vi "SR830Monitor-new2.vi"() -> ()   [LabVIEW 2016]
doc: "This VI is an example of storing and recovering data from the SR830 data buffers .\nDATA STORAGE RATE specifes the rate at which data is added to the data buffers .\nSCAN LENGTH specifies the approximate length of the data acquisition scan is seconds .\nPLOT GRAPH, PLOT CH 1 DATA and PLOT CH 2 DATA specify if the respective graphs will be displayed .\nAfter data storage is completed , the channel 1 and channel 2 points are downloaded from the instrument to the CH 1 POINTS and CH 2 POINTS arrays respectively . \nSince data recovered (using the SR830 receive message.vi) is in the string format , this VI requires a considerable amount of time to format the data into an array of floating point numbers . A quicker way would be to store the string in a file and use a CIN to speed up the process ."
uses:
  Global/Global Variables/Data_Display_global.vi
  Instrument_Setup.vi
  Utility/Monitor Communication/sub-vis/SR830_Open_Queue.vi
  Utility/Monitor Communication/sub-vis/SR830_Check_Queue.vi
  Utility/Monitor Communication/SR830/SR830-Cluster.ctl
panel:
  out "SR830":T1={"Lockin 1"=[], "X1"=0.0, "Y1"=0.0, "X1 Percent"=0.0, "X1 Overload"=FALSE, "Y1 Overload"=FALSE, "Unit X1"="nV", "Unit X2"="nV", "Unit X2a"="nV", "Unit X1a"="nV", "Sensitivity Setpoint"=26, "X1 Percent 2"=0.0} {"X1 Percent 2" scale=0.0..1.0; "Sensitivity Setpoint" items=["2 nV", "5 nV", "10 nV", "20 nV", "50 nV", "100 nV", "200 nV", "500 nV", "1 µV", "2 µV", "5 µV", "10 µV", "20 µV", "50 µV", "100 µV", "200 µV", "500 µV", "1 mV", "2 mV", "5 mV", "10 mV", "20 mV", "50 mV", "100 mV", "200 mV", "500 mV", "1 V", ""]; "X1 Percent" scale=0.0..1.0; "X1" format="%#4_5f"}
  in  "Stopp":bool
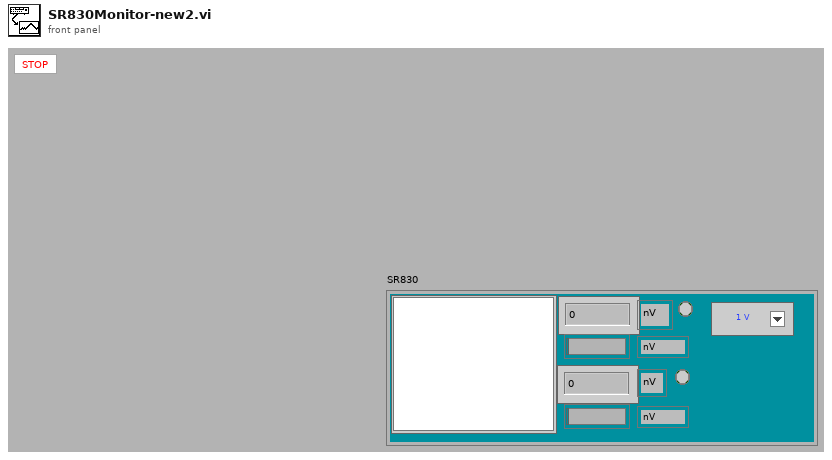
[diagram p1: front panel]
types:
  T1 = typedef "SR830-Cluster.ctl" = cluster{"Lockin 1":dbl[][], "X1":dbl, "Y1":dbl, "X1 Percent":dbl, "X1 Overload":bool, "Y1 Overload":bool, "Unit X1":string, "Unit X2":string, "Unit X2a":string, "Unit X1a":string, "Sensitivity Setpoint":i16, "X1 Percent 2":dbl}
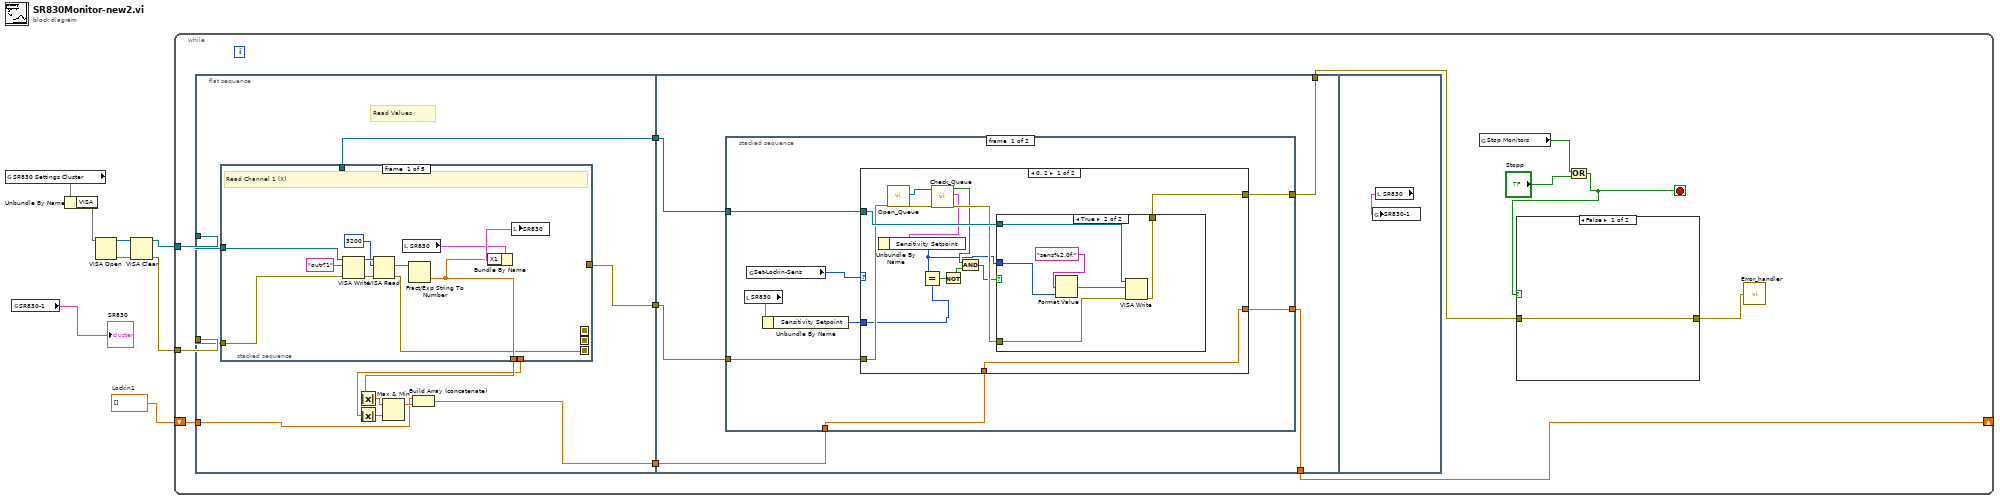
[diagram p0: block diagram]
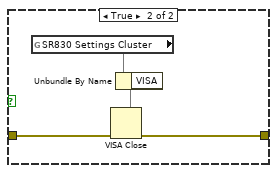
[diagram p2: hidden frame]
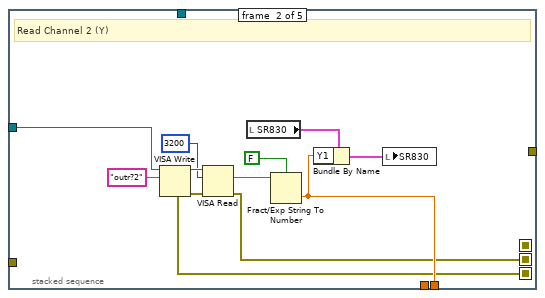
[diagram p3: hidden frame]
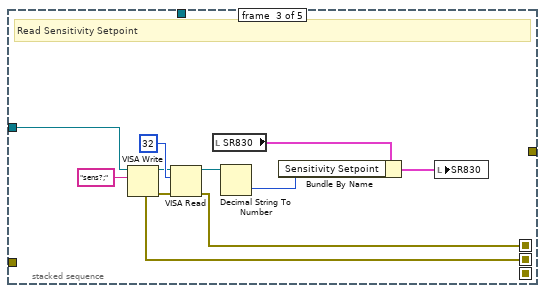
[diagram p4: hidden frame]
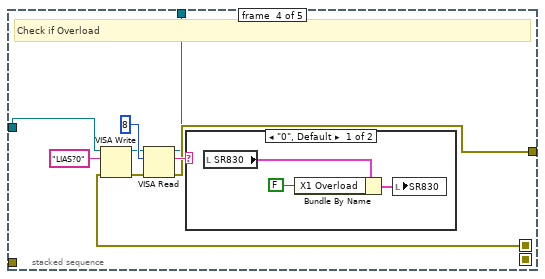
[diagram p5: hidden frame]
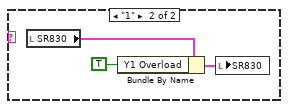
[diagram p6: hidden frame]
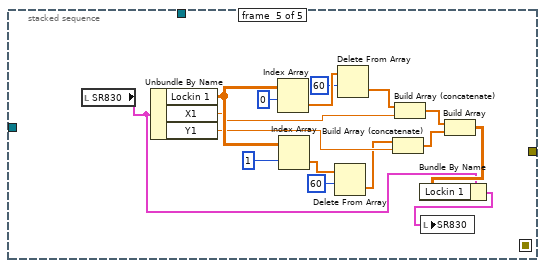
[diagram p7: hidden frame]
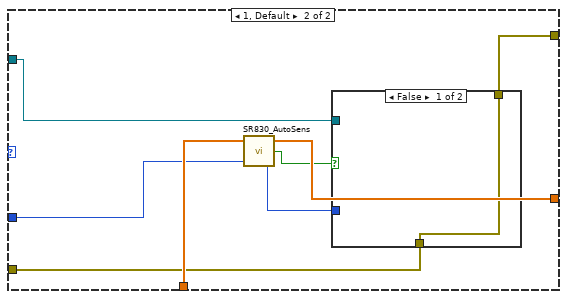
[diagram p9: hidden frame]
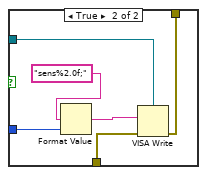
[diagram p10: hidden frame]
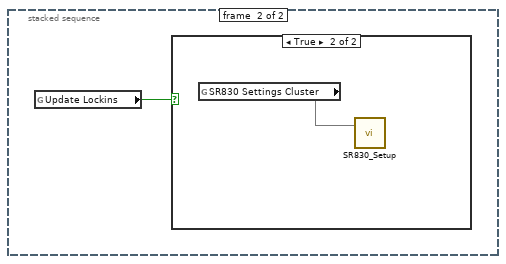
[diagram p11: hidden frame]
diagram:
  w7 = dbl[] []  # Lockin1
  n1 = global read "Instrument_Setup.vi" "SR830 Settings Cluster"() -> (w2)
  n2 = global read "Data_Display_global.vi" "SR830-1"() -> (→"SR830":T1)
  n3 = Unbundle By Name(w2) -> ("VISA"=w1)
  n4 = VISA Open(VISA resource name=w1) -> (VISA resource name=w5:refnum<visa-resource-name>, error out=w6:errorcluster)  [unwired: 4 in]
  n5 = VISA Clear(VISA resource name=w5, error in (no error)=w6) -> (VISA resource name out=w4:refnum<visa-resource-name>, error out=w3:errorcluster)
  n6 = while {
    tunnel: w4 -> [w17]
    tunnel: w3 -> [w16]
    shift-right: [w12] -> _
    shift-left: w7 -> [w18]
    stop <- w11 stop-if-true
    n7 = flat-sequence {
      tunnel: w18 -> [w31]
      tunnel: w17 -> [w29]
      tunnel: w16 -> [w28]
      tunnel: [w27] -> w15
      tunnel: [w30] -> w14
      tunnel: [w26] -> w13
      tunnel: w15 -> [w105]
      tunnel: w14 -> [w106]
      tunnel: w13 -> [w104]
      tunnel: [w103] -> w12
      tunnel: [w102] -> w10
      frame #0 {
        # "Read Values"
        n8 = stacked-sequence {
          seq-local: [w39 _ _ _ _] -> [_ w50 _ _ _]
          seq-local: [_ w49 _ _ _] -> [_ _ w61 _ _]
          seq-local: [_ _ w60 _ _] -> [_ _ _ w73 _]
          tunnel: [w41 _ _ _ _] -> w34
          tunnel: [_ w51 _ _ _] -> w33
          tunnel: w29 -> [w38 w48 w63 w76 _]
          tunnel: w28 -> [w40 _ _ _ _]
          tunnel: [_ _ _ w72 _] -> w27
          tunnel: [_ _ _ w71 _] -> w26
          frame #0 {
            # "Read Channel 1 (X)"
            n9 = VISA Write(VISA resource name=w38, write buffer="outr?1", error in (no error)=w40) -> (VISA resource name out=w45:refnum<visa-resource-name>, error out=w46:errorcluster)  [unwired: 1 out]
            n10 = VISA Read(VISA resource name=w45, byte count=3200, error in (no error)=w46) -> (read buffer=w43:string, error out=w39:errorcluster)  [unwired: 2 out]
            n11 = local read "SR830"() -> (w37:T1)
            n12 = Fract/Exp String To Number(string=w43) -> (number=w41:dbl)  [unwired: 3 in, 1 out]
            n13 = Bundle By Name(cluster=w37, "X1"=w41) -> (w42:T1)
            n14 = local write "SR830"(w42) -> ()
          }
          frame #1 {
            # "Read Channel 2 (Y)"
            n15 = VISA Write(VISA resource name=w48, write buffer="outr?2", error in (no error)=w50) -> (VISA resource name out=w57:refnum<visa-resource-name>, error out=w58:errorcluster)  [unwired: 1 out]
            n16 = VISA Read(VISA resource name=w57, byte count=3200, error in (no error)=w58) -> (read buffer=w52:string, error out=w49:errorcluster)  [unwired: 2 out]
            n17 = local read "SR830"() -> (w54:T1)
            n18 = Fract/Exp String To Number(use system decimal point (T)=FALSE, string=w52) -> (number=w51:dbl)  [unwired: 2 in, 1 out]
            n19 = Bundle By Name(cluster=w54, "Y1"=w51) -> (w55:T1)
            n20 = local write "SR830"(w55) -> ()
          }
          frame #2 {
            # "Read Sensitivity Setpoint"
            n21 = VISA Write(VISA resource name=w63, write buffer="sens?;", error in (no error)=w61) -> (VISA resource name out=w62:refnum<visa-resource-name>, error out=w69:errorcluster)  [unwired: 1 out]
            n22 = VISA Read(VISA resource name=w62, byte count=32, error in (no error)=w69) -> (VISA resource name out=w67:refnum<visa-resource-name>, error out=w60:errorcluster)  [unwired: 2 out]
            n23 = local read "SR830"() -> (w66:T1)
            n24 = Decimal String To Number(string=w67) -> (number=w64:i32)  [unwired: 2 in, 1 out]
            n25 = Bundle By Name(cluster=w66, "Sensitivity Setpoint"=w64) -> (w65:T1)
            n26 = local write "SR830"(w65) -> ()
          }
          frame #3 {
            # "Check if Overload"
            n27 = VISA Write(VISA resource name=w76, write buffer="LIAS?0", error in (no error)=w73) -> (VISA resource name out=w74:refnum<visa-resource-name>, error out=w79:errorcluster)  [unwired: 1 out]
            n28 = VISA Read(VISA resource name=w74, byte count=8, error in (no error)=w79) -> (VISA resource name out=w71:refnum<visa-resource-name>, read buffer=w75:string, error out=w72:errorcluster)  [unwired: 1 out]
            n29 = case shown="\"0\", Default" w75 {
              frame "0", Default {
                n30 = local read "SR830"() -> (w82:T1)
                n31 = Bundle By Name(cluster=w82, "X1 Overload"=FALSE) -> (w81:T1)
                n32 = local write "SR830"(w81) -> ()
              }
              frame "1" {
                n33 = local read "SR830"() -> (w85:T1)
                n34 = Bundle By Name(cluster=w85, "Y1 Overload"=TRUE) -> (w84:T1)
                n35 = local write "SR830"(w84) -> ()
              }
            }
          }
          frame #4 {
            n36 = local read "SR830"() -> (w87:T1)
            n37 = Unbundle By Name(w87) -> ("Lockin 1"=w101:dbl[][], "X1"=w98:dbl, "Y1"=w97:dbl)
            n38 = Index Array(array=w101, index (row)=0) -> (element=w94:dbl[])  [unwired: 1 in]
            n39 = Index Array(array=w101, index (row)=1) -> (element=w92:dbl[])  [unwired: 1 in]
            n40 = Delete From Array(array=w92, length=60) -> (deleted portion=w91:dbl[])  [unwired: 1 in, 1 out]
            n41 = Delete From Array(array=w94, length=60) -> (deleted portion=w93:dbl[])  [unwired: 1 in, 1 out]
            n42 = Build Array (concatenate)(w91, w97) -> (w96:dbl[])
            n43 = Build Array (concatenate)(w93, w98) -> (w95:dbl[])
            n44 = Build Array(w95, w96) -> (w88:dbl[][])
            n45 = Bundle By Name(cluster=w87, "Lockin 1"=w88) -> (w86:T1)
            n46 = local write "SR830"(w86) -> ()
          }
        }
        n47 = Absolute Value(x=w34) -> (abs(x)=w36:dbl)
        n48 = Absolute Value(x=w33) -> (abs(x)=w35:dbl)
        n49 = Max & Min(x=w36, y=w35) -> (max(x,y)=w32:dbl)  [unwired: 1 out]
        n50 = Build Array (concatenate)(w31, w32) -> (w30:dbl[])
      }
      frame #1 {
        n51 = stacked-sequence {
          tunnel: [w109 _] -> w103
          tunnel: w106 -> [w110 _]
          tunnel: w105 -> [w113 _]
          tunnel: w104 -> [w112 _]
          tunnel: [w111 _] -> w102
          frame #0 {
            n52 = local read "SR830"() -> (w108:T1)
            n53 = global read "Instrument_Setup.vi" "Set-Lockin-Sens"() -> (w114:u16)
            n54 = Unbundle By Name(w108) -> ("Sensitivity Setpoint"=w107:i16)
            n55 = case shown="0, 2" w114 {
              tunnel: w113 -> [w125 w137]
              tunnel: w112 -> [w128 w139]
              tunnel: [w118 w136] -> w111
              tunnel: w110 -> [w117 w143]
              tunnel: [w117 w142] -> w109
              tunnel: w107 -> [w116 w141]
              frame 0, 2 {
                n56 = call-poly "Open_Queue.vi"("error in (no error)"=w125) -> ("error out"=w126:errorcluster, "queue out"=w127:refnum<queue>)  [unwired: 9 in]
                n57 = call-poly "Check_Queue.vi"("error in (no error)"=w126, "queue"=w127) -> ("error out"=w124:errorcluster, "SR830"=w123:T1, "New Entries?"=w120:bool)  [unwired: 6 in]
                n58 = Unbundle By Name(w123) -> ("Sensitivity Setpoint"=w115:i16)
                n59 = Equal?(x=w115, y=w116) -> (x = y?=w122:bool)
                n60 = Not(x=w122) -> (.not. x?=w121:bool)
                n61 = And(x=w120, y=w121) -> (x .and. y?=w119:bool)
                n62 = case shown="True" w119 {
                  tunnel: w115 -> [_ w135]
                  tunnel: [w129 w134] -> w118
                  tunnel: w124 -> [w129 w131]
                  tunnel: w128 -> [_ w130]
                  frame False {
                  }
                  frame True {
                    n63 = Format Value(format string="sens%2.0f;", value (0)=w135) -> (output string=w133:string)  [unwired: 1 in]
                    n64 = VISA Write(VISA resource name=w130, write buffer=w133, error in (no error)=w131) -> (error out=w134:errorcluster)  [unwired: 2 out]
                  }
                }
              }
              frame 1, Default {
                n65 = call "SR830_AutoSens.vi"("Sensitivity"=w141, "Data in"=w143) -> ("Sensitivity Out"=w138:i32, "Set Sensitivity"=w140:bool, "Data out"=w142:dbl[])  [unwired: 1 in]
                n66 = case shown="False" w140 {
                  tunnel: w139 -> [_ w148]
                  tunnel: w138 -> [_ w147]
                  tunnel: w137 -> [w144 w146]
                  tunnel: [w144 w145] -> w136
                  frame False {
                  }
                  frame True {
                    n67 = Format Value(format string="sens%2.0f;", value (0)=w147) -> (output string=w150:string)  [unwired: 1 in]
                    n68 = VISA Write(VISA resource name=w148, write buffer=w150, error in (no error)=w146) -> (error out=w145:errorcluster)  [unwired: 2 out]
                  }
                }
              }
            }
          }
          frame #1 {
            n69 = global read "Instrument_Setup.vi" "Update Lockins"() -> (w151:bool)
            n70 = case shown="True" w151 {
              frame False {
              }
              frame True {
                n71 = global read "Instrument_Setup.vi" "SR830 Settings Cluster"() -> (w152)
                n72 = call "SR830_Setup.vi"("SR830 Settings Cluster"=w152) -> ()  [unwired: 2 in]
              }
            }
          }
        }
      }
      frame #2 {
        n73 = local read "SR830"() -> (w153:T1)
        n74 = global write "Data_Display_global.vi" "SR830-1"(w153) -> ()
      }
    }
    n75 = global read "Data_Display_global.vi" "Stop Monitors"() -> (w20:bool)
    n76 = Or(x=w20, y="Stopp") -> (x .or. y?=w11:bool)
    n77 = case shown="False" w11 {
      tunnel: w10 -> [w21 w23]
      tunnel: [w21 w22] -> w9
      frame False {
      }
      frame True {
        n78 = global read "Instrument_Setup.vi" "SR830 Settings Cluster"() -> (w25)
        n79 = Unbundle By Name(w25) -> ("VISA"=w24)
        n80 = VISA Close(VISA resource name=w24, error in (no error)=w23) -> (error out=w22:errorcluster)
      }
    }
    n81 = call "Error_handler.vi"("error constant"=w9) -> ()
  }
